vi "Tree_Go to next displayed item.vi"(7 "Direction":enum16{"Down", "Up"}(ring), 11 "Tree ref":refnum<vi>) -> ()   [LabVIEW 2023]
doc: "On kep up or down, go to next displayed item in list. Assume that keyboard navigation is in use, and replace the last selected item. THis will probably fila is multiple items are already selected, and so should be disabled if that's the case."
panel:
  out "first item":bool
  out "last item":bool
  out "error out":errorcluster
  in  "Tree":string[](tree)
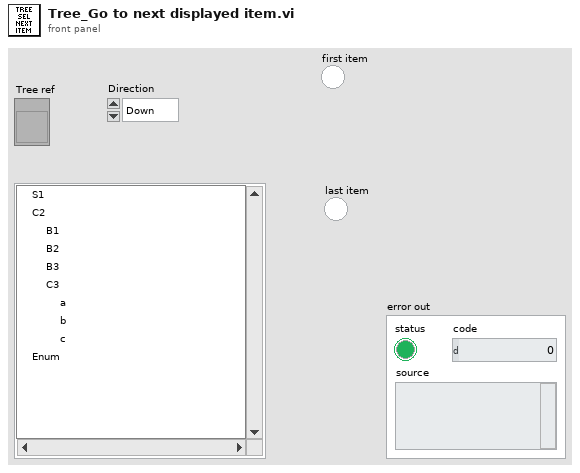
[diagram p1: front panel]
types:
  T1 = enum16{"Unknown", "Base", "Scripting", "Private", "Deprecated", "None", "Divider"}
  T2 = cluster{"Index":u16, "Property Type":enum16{"Unknown", "Base", "Scripting", "Private", "Deprecated", "None", "Divider"}, "ID String":string, "Dotted ID String":string, "Class":string, "Parent":string, "Display name full":string, "Display name short":string, "Parents Array":string[], "Indent":u16}
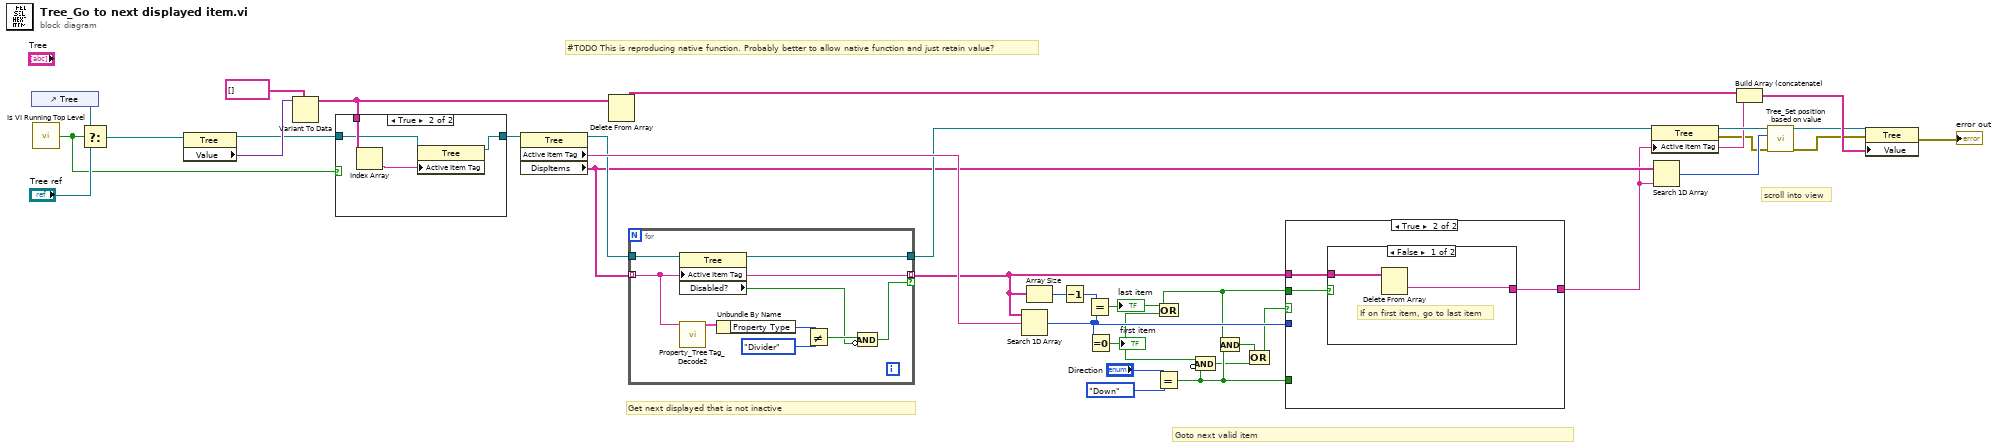
[diagram p0: block diagram]
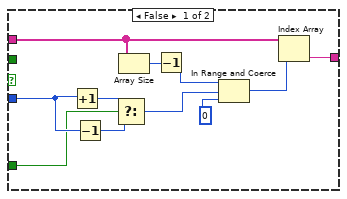
[diagram p3: hidden frame]
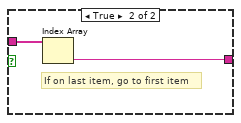
[diagram p4: hidden frame]
diagram:
  # "scroll into view"
  # "#TODO This is reproducing native function. Probably better to allow native function and just retain value?"
  # "Goto next valid item"
  # "Get next displayed that is not inactive"
  n1 = control-ref of="Tree"() -> (w34:refnum<vi>)
  n2 = call "Is VI Running Top Level.vi"() -> ("Top Level?"=w18:bool)  [unwired: 5 in]
  n3 = Select(t=w34, s=w18, f="Tree ref") -> (s? t:f=w24:refnum<vi>)
  n4 = property class="Tree"(reference=w24) -> (reference out=w20:refnum<vi>, "Value"=w21:variant)  [unwired: 1 in, 1 out]
  n5 = Variant To Data(type=string[] [] ("Active Item:Tag"), Variant=w21) -> (data=w23:string[])  [unwired: 1 in, 1 out]
  n6 = case shown="True" w18 {
    tunnel: w23 -> [_ w39]
    tunnel: w20 -> [w35 w37]
    tunnel: [w35 w36] -> w19
    frame False {
    }
    frame True {
      n7 = Index Array(array=w39) -> (element=w38:string)  [unwired: 1 in]
      n8 = property class="Tree"(reference=w37, "Active Item Tag"=w38) -> (reference out=w36:refnum<vi>)  [unwired: 1 in, 1 out]
    }
  }
  n9 = property class="Tree"(reference=w19) -> (reference out=w27:refnum<vi>, "Active Item Tag"=w28:string, "DispItems"=w15:string[])  [unwired: 1 in, 1 out]
  n10 = Delete From Array(array=w23) -> (array with subset deleted=w29:string[])  [unwired: 2 in, 1 out]
  n11 = for {
    tunnel: w27 -> [w48]
    tunnel: [w47] -> w25 mode=indexing if=w41
    tunnel: w15 -> [w47] mode=indexing
    tunnel: [w43] -> w26
    n12 = property class="Tree"(reference=w48, "Active Item Tag"=w47) -> (reference out=w43:refnum<vi>, "Disabled?"=w40:bool)  [unwired: 1 in, 1 out]
    n13 = call "Property_Tree Tag_Decode2.vi"("Tag In"=w47) -> ("TagData"=w46:T2)  [unwired: 10 in]
    n14 = Unbundle By Name(w46) -> ("Property Type"=w45:T1)
    n15 = Not Equal?(x=w45, y=T1."Divider" ("Property Type")) -> (x != y?=w42:bool)
    n16 = Compound Arithmetic op=AND(w42, invert w40) -> (w41:bool)
  }
  n17 = Search 1D Array(1D array=w25, element=w28) -> (index of element=w7:i32)  [unwired: 1 in]
  n18 = Array Size(array=w25) -> (size(s)=w9:i32)
  n19 = Decrement(x=w9) -> (x-1=w8:i32)
  n20 = Equal?(x=w8, y=w7) -> (x = y?=w6:bool)
  "last item" <- w6
  n21 = Equal To 0?(x=w7) -> (x = 0?=w5:bool)
  "first item" <- w5
  n22 = Equal?(x="Direction", y=enum16{"Down", "Up"}."Down" ("Direction")) -> (x = y?=w4:bool)
  n23 = Compound Arithmetic op=OR(w6, w5) -> ()  [unwired: 1 out]
  n24 = Compound Arithmetic op=AND(w5, invert w4) -> (w2:bool)
  n25 = Compound Arithmetic op=AND(w6, w4) -> (w3:bool)
  n26 = Compound Arithmetic op=OR(w3, w2) -> (w1:bool)
  n27 = case shown="True" w1 {
    tunnel: [w59 w61] -> w14
    tunnel: w25 -> [w58 w62]
    tunnel: w7 -> [w57 _]
    tunnel: w4 -> [w49 _]
    tunnel: w6 -> [_ w60]
    frame False {
      n28 = Increment(x=w57) -> (x+1=w56:i32)
      n29 = Decrement(x=w57) -> (x-1=w55:i32)
      n30 = Select(t=w56, s=w49, f=w55) -> (s? t:f=w54:i32)
      n31 = Array Size(array=w58) -> (size(s)=w53:i32)
      n32 = Decrement(x=w53) -> (x-1=w50:i32)
      n33 = In Range and Coerce(upper limit=w50, x=w54, lower limit=0) -> (coerced(x)=w51:i32)  [unwired: 1 out]
      n34 = Index Array(array=w58, index=w51) -> (element=w59:string)
    }
    frame True {
      n35 = case shown="False" w60 {
        tunnel: w62 -> [w64 w66]
        tunnel: [w63 w65] -> w61
        frame False {
          # "If on first item, go to last item"
          n36 = Delete From Array(array=w64) -> (deleted portion=w63:string)  [unwired: 2 in, 1 out]
        }
        frame True {
          # "If on last item, go to first item"
          n37 = Index Array(array=w66) -> (element=w65:string)  [unwired: 1 in]
        }
      }
    }
  }
  n38 = property class="Tree"(reference=w26, "Active Item Tag"=w14) -> (reference out=w17:refnum<vi>, error out=w12:errorcluster)  [unwired: 1 in]
  n39 = Search 1D Array(1D array=w15, element=w14) -> (index of element=w13:i32)  [unwired: 1 in]
  n40 = Build Array (concatenate)(w29, w14) -> (w30:string[])
  n41 = call "Tree_Set position based on value.vi"("error in (no error)"=w12, "Selected Row"=w13, "Tree Ref"=w17) -> ("error out"=w11:errorcluster, "Tree Ref"=w16:refnum<vi>)  [unwired: 7 in]
  n42 = property class="Tree"(reference=w16, error in=w11, "Value"=w30) -> (error out=→"error out":errorcluster)  [unwired: 1 out]
